vi "end_tag.vi"(1 "content":string, 2 "tag":string) -> (0 "full command":string)   [LabVIEW 2014]
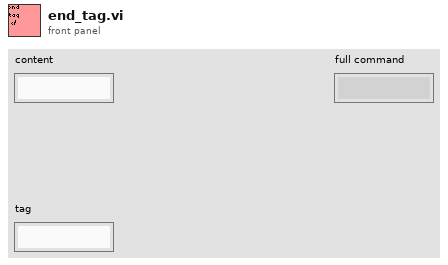
[diagram p1: front panel]
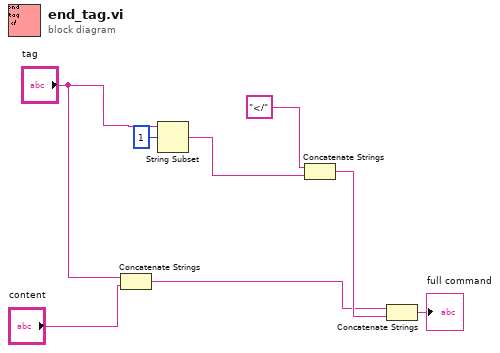
[diagram p0: block diagram]
diagram:
  n1 = Concatenate Strings("tag", "content") -> (w3:string)
  n2 = String Subset(string="tag", offset (0)=1) -> (substring=w7:string)  [unwired: 1 in]
  n3 = Concatenate Strings("</" ("string"), w7) -> (w5:string)
  n4 = Concatenate Strings(w3, w5) -> (→"full command":string)
